vi "Send Email with Attachment LV2012 NIVerified.vi"() -> ()   [LabVIEW 2016]
uses:
  <vilib>/smtpClient/Set Message Text.vi
  <vilib>/smtpClient/LabVIEWSMTPClient.lvlib
panel:
  in  "Attachment Path":path
  in  "From: (email@site.com)":string
  in  "Port":i32=25
  in  "SMTP Outgoing Mail Server":string
  in  "Body:":string
  in  "Subject:":string
  in  "To: (email@site.com)":string
  in  "Email Account Password":string
  in  "Email Account ID":string
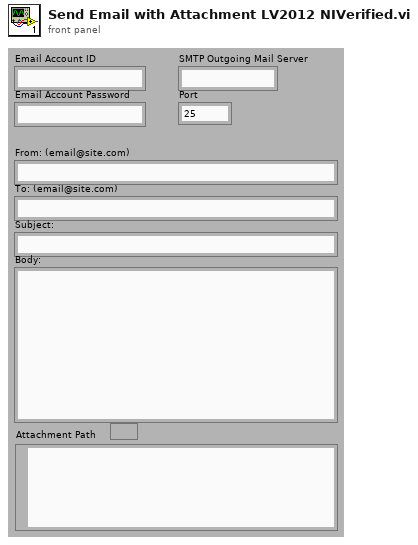
[diagram p1: front panel]
types:
  T1 = typedef "LabVIEWSMTPClient.lvlib/SmtpClientHandle.ctl" = refnum<k1>
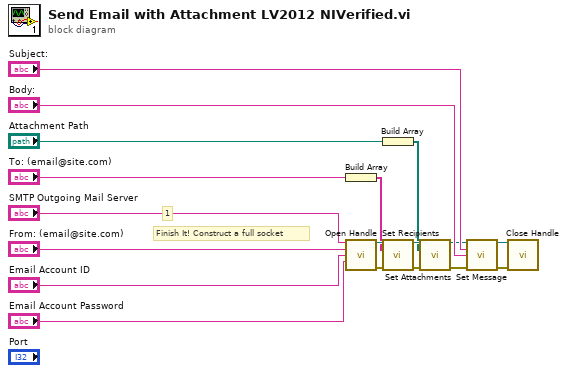
[diagram p0: block diagram]
diagram:
  # "Finish It! Construct a full socket"
  # "1"
  n1 = Build Array("To: (email@site.com)") -> (w10:string[])
  n2 = call <vilib>:"Open Handle.vi"("server address"="SMTP Outgoing Mail Server", "from"="From: (email@site.com)", "username"="Email Account ID", "password"="Email Account Password") -> ("handle out"=w18:T1, "error out"=w16:errorcluster)  [unwired: 10 in]
  n3 = Build Array("Attachment Path") -> (w6:path[])
  n4 = call <vilib>:"Set Recipients.vi"("handle in"=w18, "to"=w10, "error in (no error)"=w16) -> ("handle out"=w12:T1, "error out"=w5:errorcluster)  [unwired: 11 in]
  n5 = call <vilib>:"Set Attachments.vi"("handle in"=w12, "attachments"=w6, "error in (no error)"=w5) -> ("handle out"=w3:T1, "error out"=w2:errorcluster)  [unwired: 11 in]
  n6 = call-poly <vilib>:"Set Message.vi"("handle in"=w3, "subject"="Subject:", "plain text message"="Body:", "error in (no error)"=w2) -> ("handle out"=w4:T1, "error out"=w1:errorcluster)  [unwired: 10 in]
  n7 = call <vilib>:"Close Handle.vi"("handle in"=w4, "error in (no error)"=w1) -> ()  [unwired: 12 in, 2 out]
